vi "sensordata.vi"() -> ()   [LabVIEW 2020]
doc: "This global variable contains sensor readings."
panel:
  out "Recent_Yaw_Rate_Change (deg/s)":dbl
  out "Swerve_Recent_Velocity_Change (ft/s)":dbl
  out "Robot_Y_Odometry_Only (in)":dbl
  out "Robot_X_Odometry_Only (in)":dbl
  out "Robot_Yaw_Rate (deg/s)":dbl
  out "Vision_Fault":bool
  out "Targeting_Predictions":dbl[](array[numeric])
  out "Swerve_Ground_Velocity_Heading (deg) [0,360]":dbl
  out "Pointing_Angle_Error (deg)":dbl
  out "Swerve_Ground_Speed (ft/s)":dbl
  out "Fused_Heading_To_Target (deg)":dbl
  out "Time_Since_Pose_Update (ms)":u32
  out "Set_Robot_Pos":bool
  out "Set_Robot_Y (in)":dbl
  out "Set_Robot_X (in)":dbl
  out "IMU_Failure":bool
  out "Pointed_At_Target":bool
  out "Fused_Distance_To_Target (in)":dbl
  out "Vision_Valid":bool
  out "Robot_H (deg)":dbl
  out "Push_Robot_H (deg)":dbl
  out "Push_Robot_Pos":bool
  out "Push_Robot_Y (in)":dbl
  out "Push_Robot_X (in)":dbl
  out "Robot_Y (in)":dbl
  out "Robot_X (in)":dbl
  # "--robot pose--"
  # "--targeting info--"
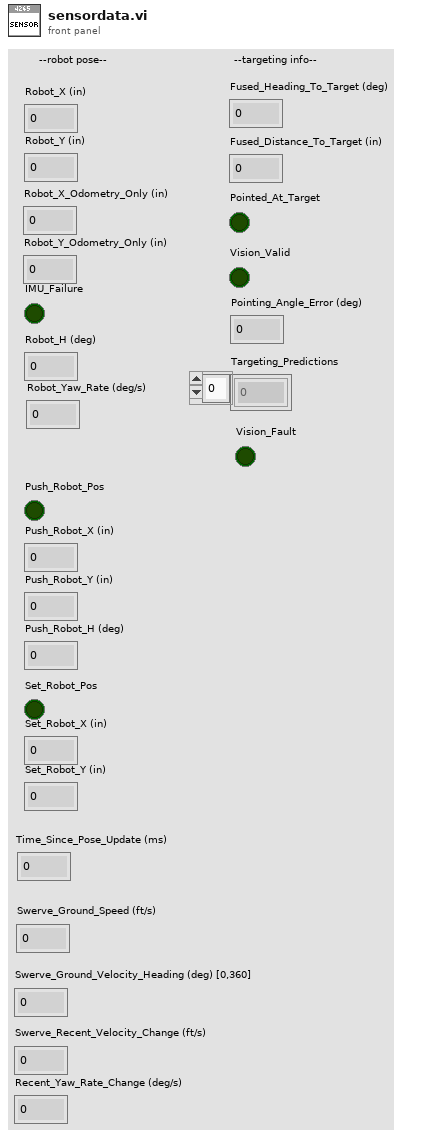
[diagram p1: front panel]
diagram:
